vi "HLine0008.vi"   [LabVIEW 2013]
uses:
  <vilib>/Heliosphere Research LLC/Advanced Plotting Toolkit/api_core/NewPlotScales.ctl
  <vilib>/Heliosphere Research LLC/Advanced Plotting Toolkit/Advanced Plotting Toolkit.lvlib
types:
  T1 = typedef "Advanced Plotting Toolkit.lvlib/NewPlotScales.ctl" = enum16{"Default", "Linear", "Log", "Symlog"}
  T2 = typedef "Advanced Plotting Toolkit.lvlib/PlotID.ctl" = i32
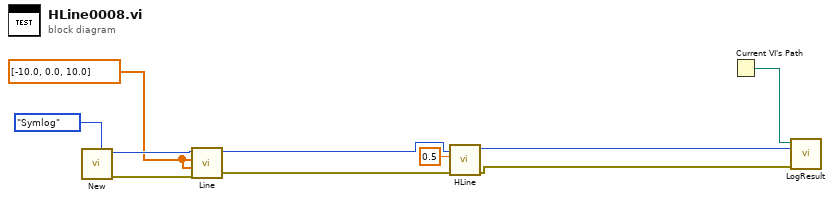
[diagram p0: block diagram]
diagram:
  w4 = dbl[] [-10.0, 0.0, 10.0] ("X Data")
  n1 = call <vilib>:"New.vi"("Y Axis Scale"=NewPlotScales."Symlog") -> ("error out"=w5:errorcluster, "Plot ID"=w6:T2)  [unwired: 9 in]
  n2 = call <vilib>:"Line.vi"("error in (no error)"=w5, "Y Data"=w4, "X Data"=w4, "Plot ID"=w6) -> ("error out"=w2:errorcluster, "Plot ID out"=w3:T2)  [unwired: 6 in]
  n3 = call <vilib>:"HLine.vi"("error in (no error)"=w2, "Y (data coords)"=0.5, "Plot ID"=w3) -> ("error out"=w7:errorcluster, "Plot ID Out"=w8:T2)  [unwired: 7 in]
  n4 = Current VI's Path() -> (path=w10:path)
  n5 = call "LogResult.vi"("Test Result"=w7, "Test Artifact"=w8, "VI Path"=w10) -> ()  [unwired: 9 in]
